vi "gps_time_frame.vi"() -> ()   [LabVIEW 2017]
uses:
  <vilib>/gmath/NI_Gmath.lvlib
panel:
  out "r 11":dbl format="%.7g"
  out "r 10":dbl format="%.7g"
  out "r 9":dbl format="%.7g"
  out "normált eredõ SNR":cluster{dbl[], dbl[]}(graph)
  out "normált X SNR (sd)":cluster{dbl[], dbl[]}(graph)
  out "normált X SNR (szum)":cluster{dbl[], dbl[]}(graph)
  out "r 8":dbl format="%.7g"
  out "r 7":dbl format="%.7g"
  out "r 6":dbl format="%.7g"
  out "r 5":dbl format="%.7g"
  out "r 4":dbl format="%.7g"
  out "r 3":dbl format="%.7g"
  out "r 2":dbl format="%.7g"
  out "r":dbl format="%.7g"
  out "impulse szum/mean":cluster{"X":dbl, "Y":dbl}[](graph)
  in  "felharmonikus N":i32=2
  in  "SNR window width [Hz]":dbl=0.2 format="%#_13g"
  in  "Case select":string(combo)="6min"
  out "impulse mean (egész jó)":cluster{"X":dbl, "Y":dbl}[](graph)
  out "impulse szum":cluster{"X":dbl, "Y":dbl}[](graph)
  out "impulse sd":cluster{"X":dbl, "Y":dbl}[](graph)
  out "impulse szum/time":cluster{"X":dbl, "Y":dbl}[](graph)
  out "X SNR (6min 0,2 Hz, 0 felharmonikus)":cluster{"X":dbl, "Y":dbl}[](graph)
  out "resultant SNR (0,2 Hz 0 felh.)":cluster{"X":dbl, "Y":dbl}[](graph)
  out "X SNR (6min 0,2 Hz, 0 felharmonikus)":cluster{"X":dbl, "Y":dbl}[](graph)
  in  "Path":path=path "C:/Users/Lenovo/Desktop/szakdoga/data/time/egyenletes_resztavok"
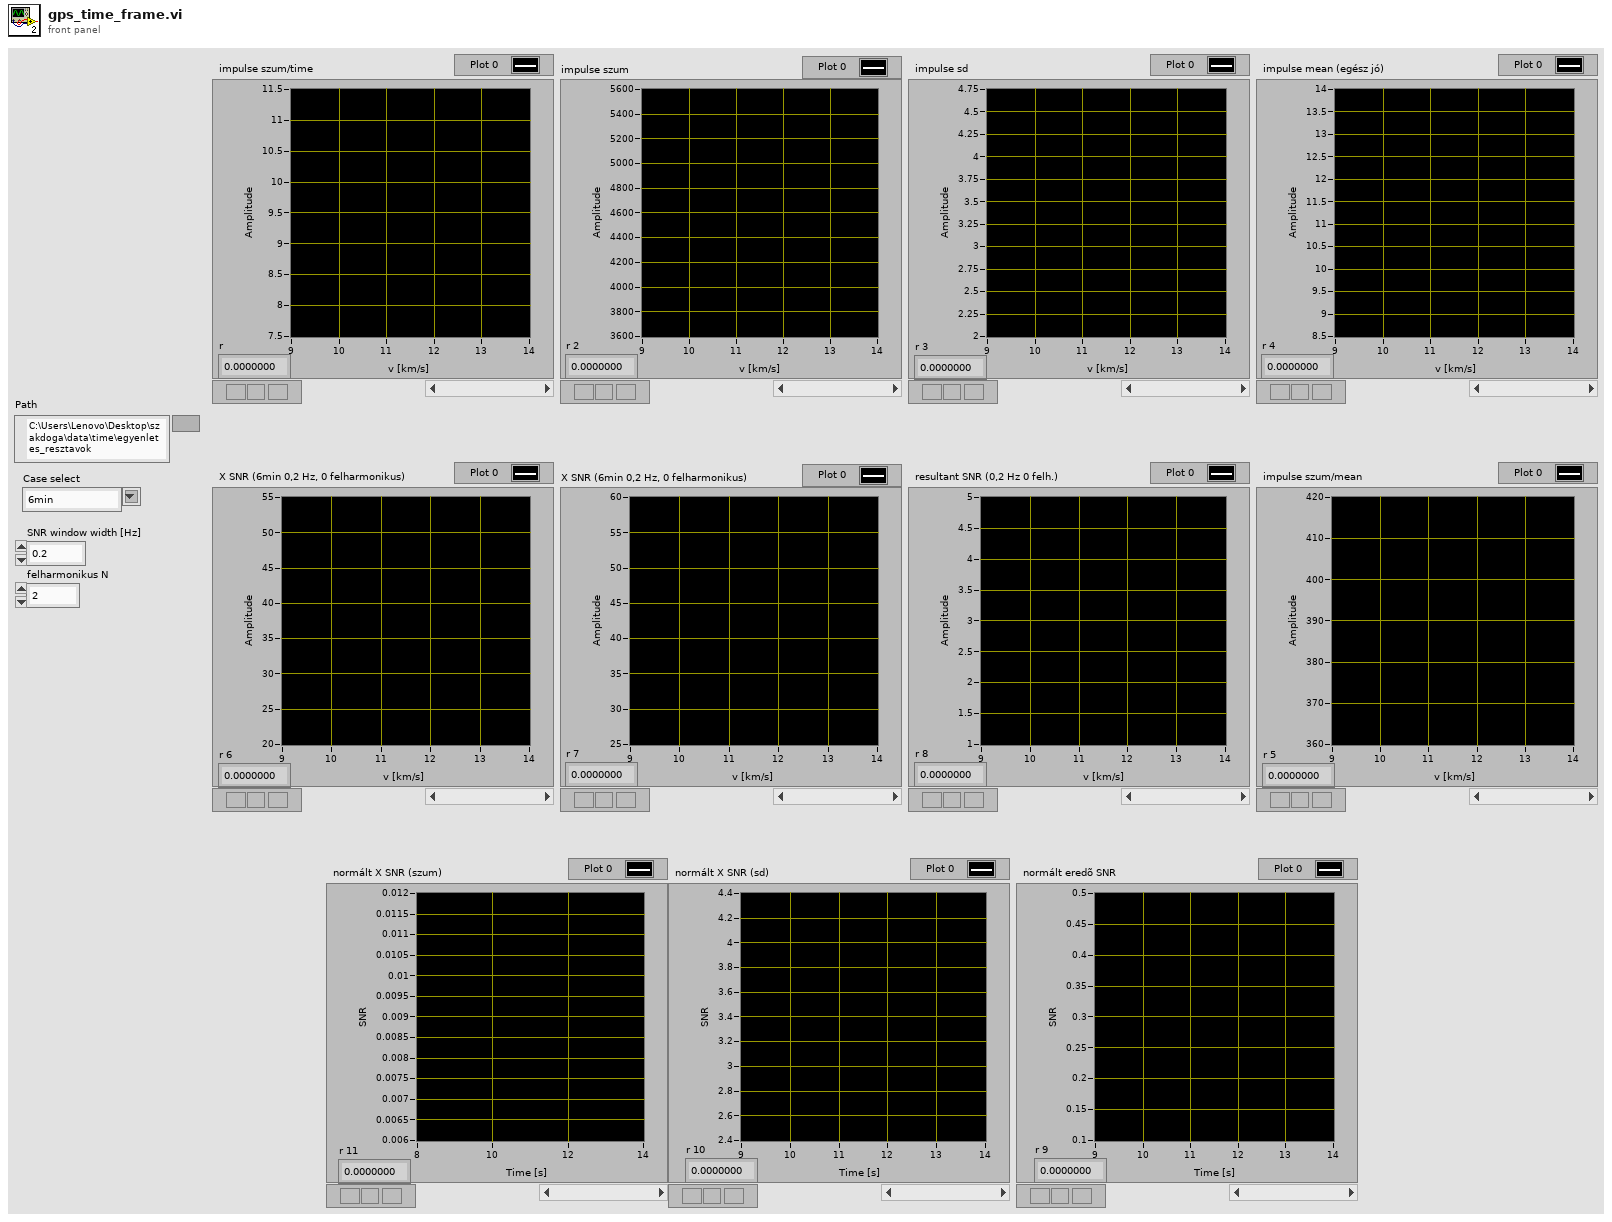
[diagram p1: front panel]
types:
  T1 = cluster{cluster{dbl, "impulse szum/time":dbl}[], cluster{dbl, "impulse  szum":dbl}[], cluster{dbl, "impulse standard deviation":dbl}[], cluster{dbl, "impulse mean":dbl}[], cluster{dbl, "X SNR 1":dbl}[], cluster{dbl, "X SNR 2":dbl}[], cluster{dbl, "X SNR 3":dbl}[], cluster{dbl, "impulse szum/avg":dbl}[]}
  T2 = cluster{cluster{dbl, dbl}[], cluster{dbl, "impulse  szum":dbl}[], cluster{dbl, "impulse standard deviation":dbl}[], cluster{dbl, "impulse mean":dbl}[], cluster{dbl, dbl}[], cluster{dbl, dbl}[], cluster{dbl, dbl}[], cluster{dbl, "impulse szum/mean":dbl}[]}
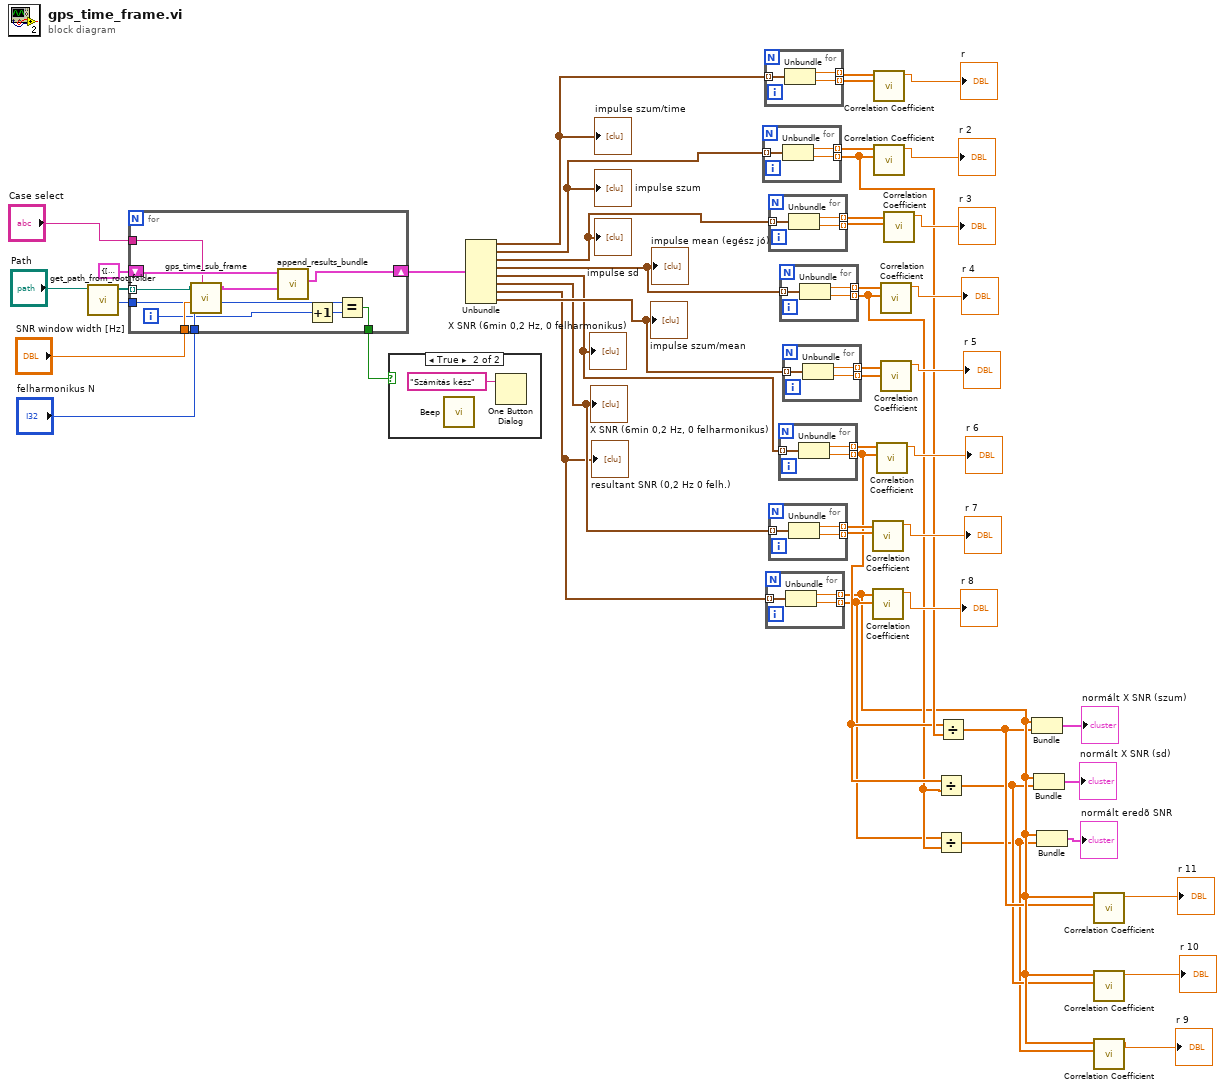
[diagram p0: block diagram]
diagram:
  n1 = call "get_path_from_root_folder.vi"("Path"="Path") -> ("Number of Files"=w45:i32, "Array"=w50:path[])  [unwired: 9 in]
  n2 = for {
    tunnel: w50 -> [w59] mode=indexing
    tunnel: "Case select" -> [w57]
    tunnel: "SNR window width [Hz]" -> [w56]
    tunnel: "felharmonikus N" -> [w55]
    tunnel: w45 -> [w54]
    tunnel: [w51] -> w44
    shift-right: [w60] -> w42
    shift-left: T1 {[], [], [], [], [], [], [], []} ("concat(X,Y)") -> [w61]
    i -> [w52]
    n3 = call "gps_time_sub_frame.vi"("Case select"=w57, "felharmonikus N"=w55, "SNR window width [Hz]"=w56, "path to binary file"=w59) -> ("output cluster"=w58:T2)  [unwired: 7 in]
    n4 = call "append_results_bundle.vi"("Y"=w58, "X"=w61) -> ("concat(X,Y)"=w60:T1)  [unwired: 8 in]
    n5 = Increment(x=w52) -> (x+1=w53:i32)
    n6 = Equal?(x=w54, y=w53) -> (x = y?=w51:bool)
  }
  n7 = case shown="True" w44 {
    frame False {
    }
    frame True {
      n8 = call <vilib>:"Beep.vi"() -> ()  [unwired: 12 in]
      n9 = One Button Dialog(message="Számítás kész") -> ()  [unwired: 1 in, 1 out]
    }
  }
  n10 = Unbundle(w42) -> (w41:cluster{dbl, "impulse szum/time":dbl}[], w40:cluster{dbl, "impulse  szum":dbl}[], w39:cluster{dbl, "impulse standard deviation":dbl}[], w38:cluster{dbl, "impulse mean":dbl}[], w36:cluster{dbl, "X SNR 1":dbl}[], w35:cluster{dbl, "X SNR 2":dbl}[], w34:cluster{dbl, "X SNR 3":dbl}[], w37:cluster{dbl, "impulse szum/avg":dbl}[])
  "X SNR (6min 0,2 Hz, 0 felharmonikus)" <- w36
  "resultant SNR (0,2 Hz 0 felh.)" <- w34
  "X SNR (6min 0,2 Hz, 0 felharmonikus)" <- w35
  "impulse szum/time" <- w41
  "impulse sd" <- w39
  "impulse szum" <- w40
  "impulse mean (egész jó)" <- w38
  "impulse szum/mean" <- w37
  n11 = for {
    tunnel: w40 -> [w65] mode=indexing
    tunnel: [w64] -> w28 mode=indexing
    tunnel: [w63] -> w11 mode=indexing
    n12 = Unbundle(w65) -> (w64:dbl, "impulse  szum"=w63:dbl)
  }
  n13 = for {
    tunnel: w41 -> [w68] mode=indexing
    tunnel: [w67] -> w33 mode=indexing
    tunnel: [w66] -> w32 mode=indexing
    n14 = Unbundle(w68) -> (w67:dbl, "impulse szum/time"=w66:dbl)
  }
  n15 = for {
    tunnel: w34 -> [w71] mode=indexing
    tunnel: [w70] -> w4 mode=indexing
    tunnel: [w69] -> w8 mode=indexing
    n16 = Unbundle(w71) -> (w70:dbl, "X SNR 3"=w69:dbl)
  }
  n17 = for {
    tunnel: w39 -> [w74] mode=indexing
    tunnel: [w73] -> w20 mode=indexing
    tunnel: [w72] -> w19 mode=indexing
    n18 = Unbundle(w74) -> (w73:dbl, "impulse standard deviation"=w72:dbl)
  }
  n19 = for {
    tunnel: w35 -> [w77] mode=indexing
    tunnel: [w76] -> w16 mode=indexing
    tunnel: [w75] -> w15 mode=indexing
    n20 = Unbundle(w77) -> (w76:dbl, "X SNR 2"=w75:dbl)
  }
  n21 = for {
    tunnel: w36 -> [w80] mode=indexing
    tunnel: [w79] -> w17 mode=indexing
    tunnel: [w78] -> w10 mode=indexing
    n22 = Unbundle(w80) -> (w79:dbl, "X SNR 1"=w78:dbl)
  }
  n23 = for {
    tunnel: w38 -> [w83] mode=indexing
    tunnel: [w82] -> w30 mode=indexing
    tunnel: [w81] -> w9 mode=indexing
    n24 = Unbundle(w83) -> (w82:dbl, "impulse mean"=w81:dbl)
  }
  n25 = for {
    tunnel: w37 -> [w86] mode=indexing
    tunnel: [w85] -> w29 mode=indexing
    tunnel: [w84] -> w18 mode=indexing
    n26 = Unbundle(w86) -> (w85:dbl, "impulse szum/avg"=w84:dbl)
  }
  n27 = call <vilib>:"Correlation Coefficient.vi"("Y"=w15, "X"=w16) -> ("correlation coefficient r"=→"r 7":dbl)  [unwired: 8 in, 1 out]
  n28 = call <vilib>:"Correlation Coefficient.vi"("Y"=w8, "X"=w4) -> ("correlation coefficient r"=→"r 8":dbl)  [unwired: 8 in, 1 out]
  n29 = call <vilib>:"Correlation Coefficient.vi"("Y"=w32, "X"=w33) -> ("correlation coefficient r"=→"r":dbl)  [unwired: 8 in, 1 out]
  n30 = call <vilib>:"Correlation Coefficient.vi"("Y"=w11, "X"=w28) -> ("correlation coefficient r"=→"r 2":dbl)  [unwired: 8 in, 1 out]
  n31 = call <vilib>:"Correlation Coefficient.vi"("Y"=w10, "X"=w17) -> ("correlation coefficient r"=→"r 6":dbl)  [unwired: 8 in, 1 out]
  n32 = call <vilib>:"Correlation Coefficient.vi"("Y"=w9, "X"=w30) -> ("correlation coefficient r"=→"r 4":dbl)  [unwired: 8 in, 1 out]
  n33 = call <vilib>:"Correlation Coefficient.vi"("Y"=w18, "X"=w29) -> ("correlation coefficient r"=→"r 5":dbl)  [unwired: 8 in, 1 out]
  n34 = call <vilib>:"Correlation Coefficient.vi"("Y"=w19, "X"=w20) -> ("correlation coefficient r"=→"r 3":dbl)  [unwired: 8 in, 1 out]
  n35 = Divide(x=w10, y=w9) -> (x/y=w2:dbl[])
  n36 = Divide(x=w8, y=w9) -> (x/y=w1:dbl[])
  n37 = Divide(x=w10, y=w11) -> (x/y=w3:dbl[])
  n38 = Bundle(w4, w3) -> (→"normált X SNR (szum)":cluster{dbl[], dbl[]})  [unwired: 1 in]
  n39 = Bundle(w4, w2) -> (→"normált X SNR (sd)":cluster{dbl[], dbl[]})  [unwired: 1 in]
  n40 = Bundle(w4, w1) -> (→"normált eredõ SNR":cluster{dbl[], dbl[]})  [unwired: 1 in]
  n41 = call <vilib>:"Correlation Coefficient.vi"("Y"=w3, "X"=w4) -> ("correlation coefficient r"=→"r 11":dbl)  [unwired: 8 in, 1 out]
  n42 = call <vilib>:"Correlation Coefficient.vi"("Y"=w2, "X"=w4) -> ("correlation coefficient r"=→"r 10":dbl)  [unwired: 8 in, 1 out]
  n43 = call <vilib>:"Correlation Coefficient.vi"("Y"=w1, "X"=w4) -> ("correlation coefficient r"=→"r 9":dbl)  [unwired: 8 in, 1 out]
